vi "compile.vi"(8 "error in (no error)":errorcluster, 11 "ScriptListCompiler in":refnum<class "ScriptListCompiler.lvclass">) -> (0 "error out":errorcluster, 3 "ScriptListCompiler out":refnum<class "ScriptListCompiler.lvclass">)   [LabVIEW 2009, in "Compiler.lvlib" / "ScriptListCompiler.lvclass"]
uses:
  ScriptListCompiler.lvclass
  ScriptListCompiler.lvclass/ScriptListCompiler.ctl
  Scripting/ScriptingEvent/ScriptEventList/ScriptEventList.lvclass
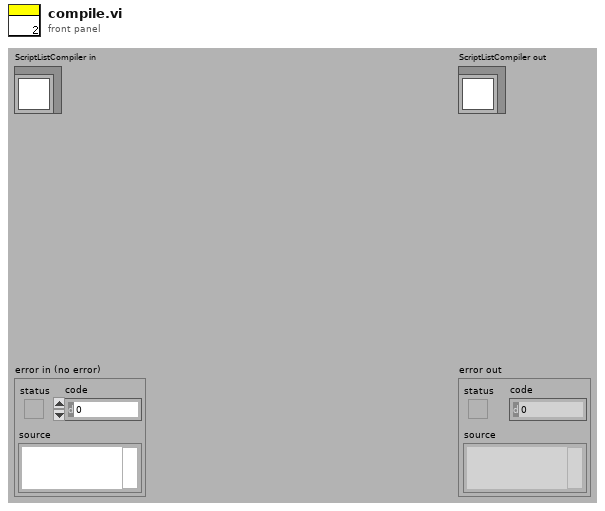
[diagram p1: front panel]
types:
  T1 = cluster{"digitalOutputList":refnum<class "ScriptEventList.lvclass">, "analogOutputList":refnum<class "ScriptEventList.lvclass">, "analogInputList":refnum<class "ScriptEventList.lvclass">, "digitalInputList":refnum<class "ScriptEventList.lvclass">, "rfOutputList":refnum<class "ScriptEventList.lvclass">}
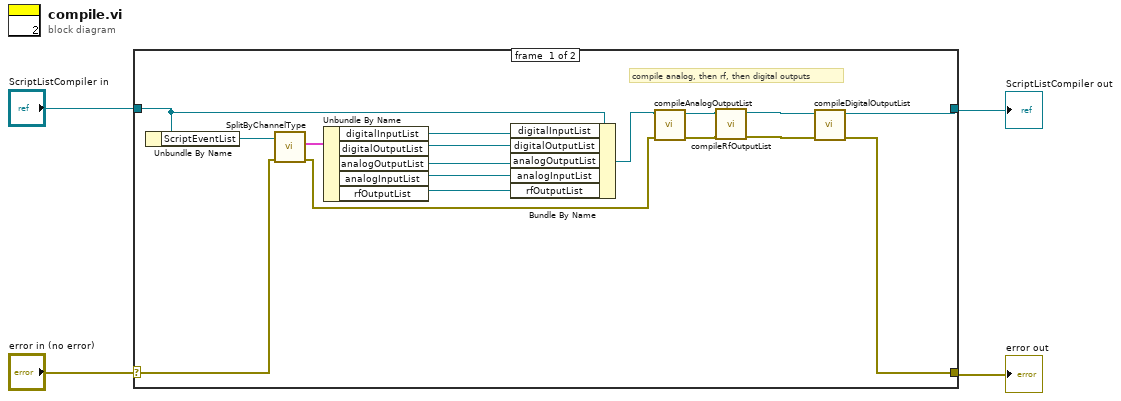
[diagram p0: block diagram]
diagram:
  n1 = case shown="No Error" "error in (no error)" {
    selector: "error in (no error)" -> [w20 w23]
    tunnel: [w15 w23] -> w3
    tunnel: [w16 w22] -> w1
    tunnel: "ScriptListCompiler in" -> [w19 w22]
    frame #0 {
      # "compile analog, then rf, then digital outputs"
      n2 = Unbundle By Name(w19) -> ("ScriptEventList"=w21:refnum<class "ScriptEventList.lvclass">)
      n3 = call "SplitByChannelType.vi"("error in (no error)"=w20, "ScriptEventList in"=w21) -> ("error out"=w17:errorcluster, "ScriptLists"=w14:T1)  [unwired: 7 in, 1 out]
      n4 = Unbundle By Name(w14) -> ("digitalInputList"=w13:refnum<class "ScriptEventList.lvclass">, "digitalOutputList"=w12:refnum<class "ScriptEventList.lvclass">, "analogOutputList"=w11:refnum<class "ScriptEventList.lvclass">, "analogInputList"=w10:refnum<class "ScriptEventList.lvclass">, "rfOutputList"=w9:refnum<class "ScriptEventList.lvclass">)
      n5 = Bundle By Name(cluster=w19, "digitalInputList"=w13, "digitalOutputList"=w12, "analogOutputList"=w11, "analogInputList"=w10, "rfOutputList"=w9) -> (w18:refnum<class "ScriptListCompiler.lvclass">)
      n6 = call "compileAnalogOutputList.vi"("error in (no error)"=w17, "ScriptListCompiler in"=w18) -> ("error out"=w7:errorcluster, "ScriptListCompiler out"=w8:refnum<class "ScriptListCompiler.lvclass">)  [unwired: 8 in]
      n7 = call "compileRfOutputList.vi"("error in (no error)"=w7, "ScriptListCompiler in"=w8) -> ("error out"=w5:errorcluster, "ScriptListCompiler out"=w6:refnum<class "ScriptListCompiler.lvclass">)  [unwired: 8 in]
      n8 = call "compileDigitalOutputList.vi"("error in (no error)"=w5, "ScriptListCompiler in"=w6) -> ("error out"=w15:errorcluster, "ScriptListCompiler out"=w16:refnum<class "ScriptListCompiler.lvclass">)  [unwired: 8 in]
    }
    frame #1 {
    }
  }
  "error out" <- w3
  "ScriptListCompiler out" <- w1
